vi "Update.vi"(8 "error in (no error)":errorcluster, 10 "Message in":refnum<class "UpdateMessage.lvclass">, 11 "Cascade in":refnum<class "Cascade.lvclass">) -> (0 "error out":errorcluster, 3 "Cascade out":refnum<class "Cascade.lvclass">)   [LabVIEW 2012, in "Cascade.lvclass"]
doc: "The update method processes the command 'update'. \n\nThe command 'update' is used for receiving new values to be set to the private data of the class. This could be seen as a public set method for setting new parameters to the private class data."
uses:
  Cascade.lvclass
  <vilib>/Distrio/Murmex/UpdateMessage/UpdateMessage.lvclass
  Cascade.lvclass/Cascade.ctl
  <vilib>/Distrio/Murmex/Murmex/Murmex.lvclass
panel:
  out "x = y?":bool
  # "This method is called when the UPDATE\ntrigger is sent. \n\nOverride this method when your component needs to\nrespond to this trigger. \n\nCall parent for proper implementation"
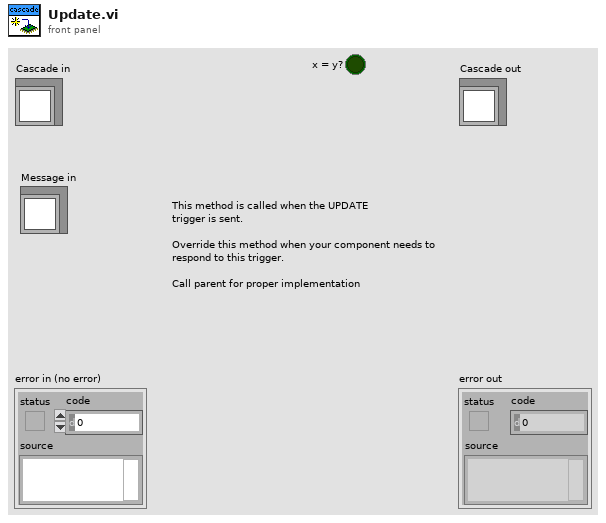
[diagram p1: front panel]
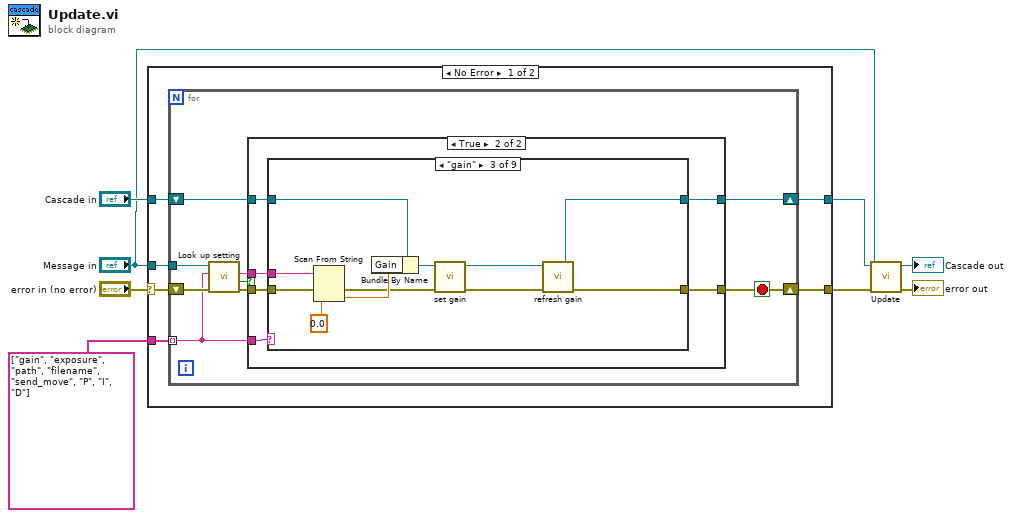
[diagram p0: block diagram]
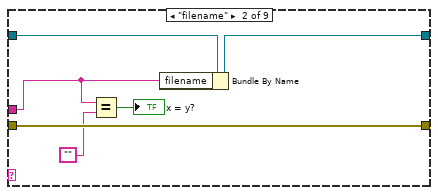
[diagram p4: hidden frame]
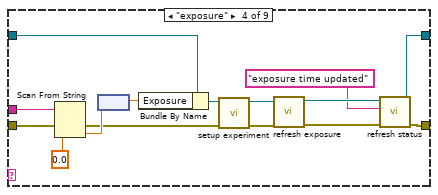
[diagram p5: hidden frame]
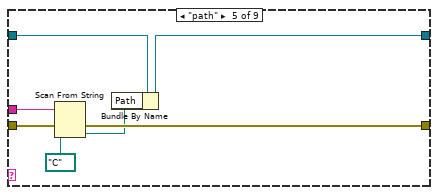
[diagram p6: hidden frame]
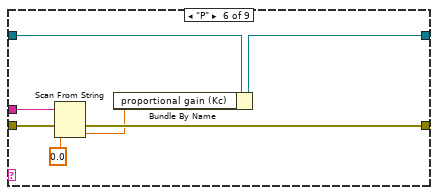
[diagram p7: hidden frame]
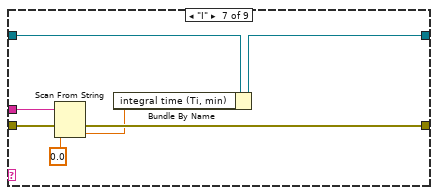
[diagram p8: hidden frame]
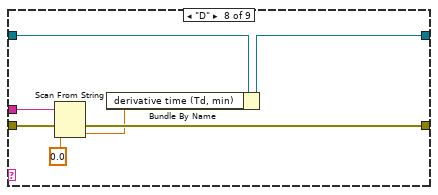
[diagram p9: hidden frame]
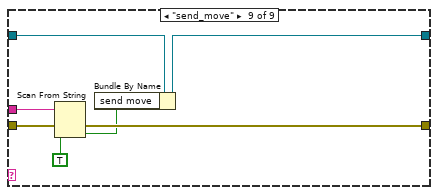
[diagram p10: hidden frame]
diagram:
  n1 = case shown="No Error" "error in (no error)" {
    selector: "error in (no error)" -> [w14 w102]
    tunnel: "Cascade in" -> [w13 w101]
    tunnel: "Message in" -> [w12 _]
    tunnel: string[] ["gain", "exposure", "path", "filename", "send_move", "P", "I", "D"] -> [w11 _]
    tunnel: [w10 w102] -> w2
    tunnel: [w9 w101] -> w1
    frame No Error {
      n2 = for {
        shift-right: [w15] -> w10
        shift-left: w14 -> [w23]
        shift-right: [w16] -> w9
        shift-left: w13 -> [w18]
        tunnel: w12 -> [w22]
        tunnel: w11 -> [w20] mode=indexing
        stop <- w15 stop-if-true
        n3 = call <vilib>:"Look up setting.vi"("error in (no error)"=w23, "tag name"=w20, "UpdateMessage in"=w22) -> ("error out"=w17:errorcluster, "found?"=w21:bool, "value"=w19:string)  [unwired: 5 in, 1 out]
        n4 = case shown="True" w21 {
          tunnel: w20 -> [_ w31]
          tunnel: w19 -> [_ w29]
          tunnel: w18 -> [w25 w28]
          tunnel: w17 -> [w24 w30]
          tunnel: [w24 w27] -> w15
          tunnel: [w25 w26] -> w16
          frame False {
          }
          frame True {
            n5 = case shown="\"gain\"" w31 {
              tunnel: w30 -> [w33 w37 w50 w65 w72 w79 w86 w93 w100]
              tunnel: w29 -> [_ w36 w49 w64 w71 w78 w85 w92 w99]
              tunnel: w28 -> [w32 w39 w48 w63 w70 w77 w84 w91 w98]
              tunnel: [w33 w37 w42 w54 w68 w75 w82 w89 w96] -> w27
              tunnel: [w32 w38 w40 w52 w69 w76 w83 w90 w97] -> w26
              frame Default {
              }
              frame "filename" {
                n6 = Equal?(x=w36, y="") -> (x = y?=→"x = y?":bool)
                n7 = Bundle By Name(cluster=w39, "filename"=w36) -> (w38:refnum<class "Cascade.lvclass">)
              }
              frame "gain" {
                n8 = Scan From String(input string=w49, error in=w50, default 1=0.0 ("settings.Gain")) -> (error out=w45:errorcluster, output 1=w47:dbl)  [unwired: 2 in, 2 out]
                n9 = Bundle By Name(cluster=w48, "Gain"=w47) -> (w44:refnum<class "Cascade.lvclass">)
                n10 = call-dynamic "set gain.vi"("error in (no error)"=w45, "Cascade in"=w44) -> ("error out"=w43:errorcluster, "Cascade out"=w41:refnum<class "Cascade.lvclass">)  [unwired: 8 in]
                n11 = call-dynamic "refresh gain.vi"("error in (no error)"=w43, "Cascade in"=w41) -> ("error out"=w42:errorcluster, "Cascade out"=w40:refnum<class "Cascade.lvclass">)  [unwired: 8 in]
              }
              frame "exposure" {
                n12 = Scan From String(input string=w64, error in=w65, default 1=0.0 ("settings.Gain")) -> (error out=w57:errorcluster, output 1=w62:dbl)  [unwired: 2 in, 2 out]
                n13 = node(w62) -> (w60:dbl[unit])
                n14 = Bundle By Name(cluster=w63, "Exposure"=w60) -> (w56:refnum<class "Cascade.lvclass">)
                n15 = call-dynamic "setup experiment.vi"("error in (no error)"=w57, "Cascade in"=w56) -> ("error out"=w59:errorcluster, "Cascade out"=w58:refnum<class "Cascade.lvclass">)  [unwired: 8 in]
                n16 = call-dynamic "refresh exposure.vi"("error in (no error)"=w59, "Cascade in"=w58) -> ("error out"=w55:errorcluster, "Cascade out"=w53:refnum<class "Cascade.lvclass">)  [unwired: 8 in]
                n17 = call-dynamic "refresh status.vi"("error in (no error)"=w55, "String In"="exposure time updated", "Cascade in"=w53) -> ("error out"=w54:errorcluster, "Cascade out"=w52:refnum<class "Cascade.lvclass">)  [unwired: 7 in]
              }
              frame "path" {
                n18 = Scan From String(input string=w71, error in=w72, default 1=path "C:/" ("settings.Path")) -> (error out=w68:errorcluster, output 1=w66:path)  [unwired: 2 in, 2 out]
                n19 = Bundle By Name(cluster=w70, "Path"=w66) -> (w69:refnum<class "Cascade.lvclass">)
              }
              frame "P" {
                n20 = Scan From String(input string=w78, error in=w79, default 1=0.0) -> (error out=w75:errorcluster, output 1=w74:dbl)  [unwired: 2 in, 2 out]
                n21 = Bundle By Name(cluster=w77, "proportional gain (Kc)"=w74) -> (w76:refnum<class "Cascade.lvclass">)
              }
              frame "I" {
                n22 = Scan From String(input string=w85, error in=w86, default 1=0.0) -> (error out=w82:errorcluster, output 1=w81:dbl)  [unwired: 2 in, 2 out]
                n23 = Bundle By Name(cluster=w84, "integral time (Ti, min)"=w81) -> (w83:refnum<class "Cascade.lvclass">)
              }
              frame "D" {
                n24 = Scan From String(input string=w92, error in=w93, default 1=0.0) -> (error out=w89:errorcluster, output 1=w88:dbl)  [unwired: 2 in, 2 out]
                n25 = Bundle By Name(cluster=w91, "derivative time (Td, min)"=w88) -> (w90:refnum<class "Cascade.lvclass">)
              }
              frame "send_move" {
                n26 = Scan From String(input string=w99, error in=w100, default 1=TRUE) -> (error out=w96:errorcluster, output 1=w94:bool)  [unwired: 2 in, 2 out]
                n27 = Bundle By Name(cluster=w98, "send move"=w94) -> (w97:refnum<class "Cascade.lvclass">)
              }
            }
          }
        }
      }
    }
    frame Error {
    }
  }
  n28 = call-parent "Update.vi"("error in (no error)"=w2, "Message in"="Message in", "Murmex in"=w1) -> ("error out"=→"error out":errorcluster, "Murmex out"=→"Cascade out":refnum<class "Cascade.lvclass">)  [unwired: 7 in]
